vi "sub_scout_logformat_convert.vi"   [LabVIEW 2019]
types:
  T1 = enum16{"read", "write utm", "write heading", "write mode"}
  T2 = cluster{"System Feedback":cluster{"system state":string, "Control Mode":u8, "Battery Voltage":dbl, "error code High":u8, "error code Low":u8}, "Motion Feedback":cluster{"Linear Velocity (m/s)":dbl, "Angular Velocity (rad/s)":dbl}}
  T3 = cluster{"system state":string, "Control Mode":u8, "Battery Voltage":dbl, "error code High":u8, "error code Low":u8}
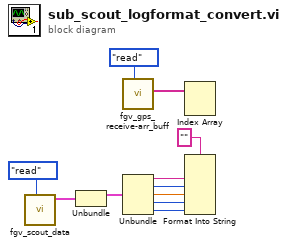
[diagram p0: block diagram]
diagram:
  n1 = call "fgv_scout_data.vi"("cmd"=enum16{"write", "read"}."read") -> ("agv data out"=w8:T2)  [unwired: 10 in]
  n2 = Unbundle(w8) -> ("System Feedback"=w9:T3)  [unwired: 1 out]
  n3 = call "fgv_gps_receive-arr_buff.vi"("cmd"=T1."read") -> ("protocol arrary"=w10:string[])  [unwired: 8 in, 2 out]
  n4 = Unbundle(w9) -> ("system state"=w3:string, "Control Mode"=w4:u8, "Battery Voltage"=w5:dbl, "error code High"=w6:u8, "error code Low"=w7:u8)
  n5 = Index Array(array=w10) -> ()  [unwired: 2 in, 2 out]
  n6 = Format Into String(format string="" ("포맷 문자열"), w3, w4, w5, w6, w7) -> ()  [unwired: 2 in, 2 out]
